vi "Untitled 11.vi"() -> ()   [LabVIEW 2017]
uses:
  <vilib>/Utility/file.llb/Read Delimited Spreadsheet (string).vi
panel:
  out "Array":string[](array[string])
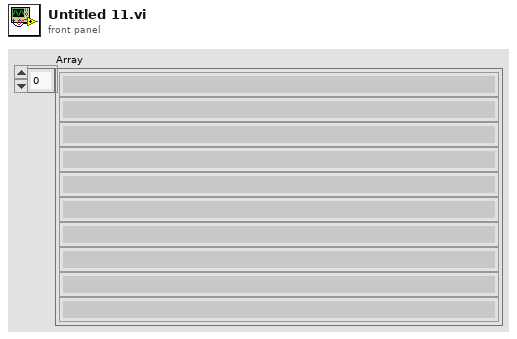
[diagram p1: front panel]
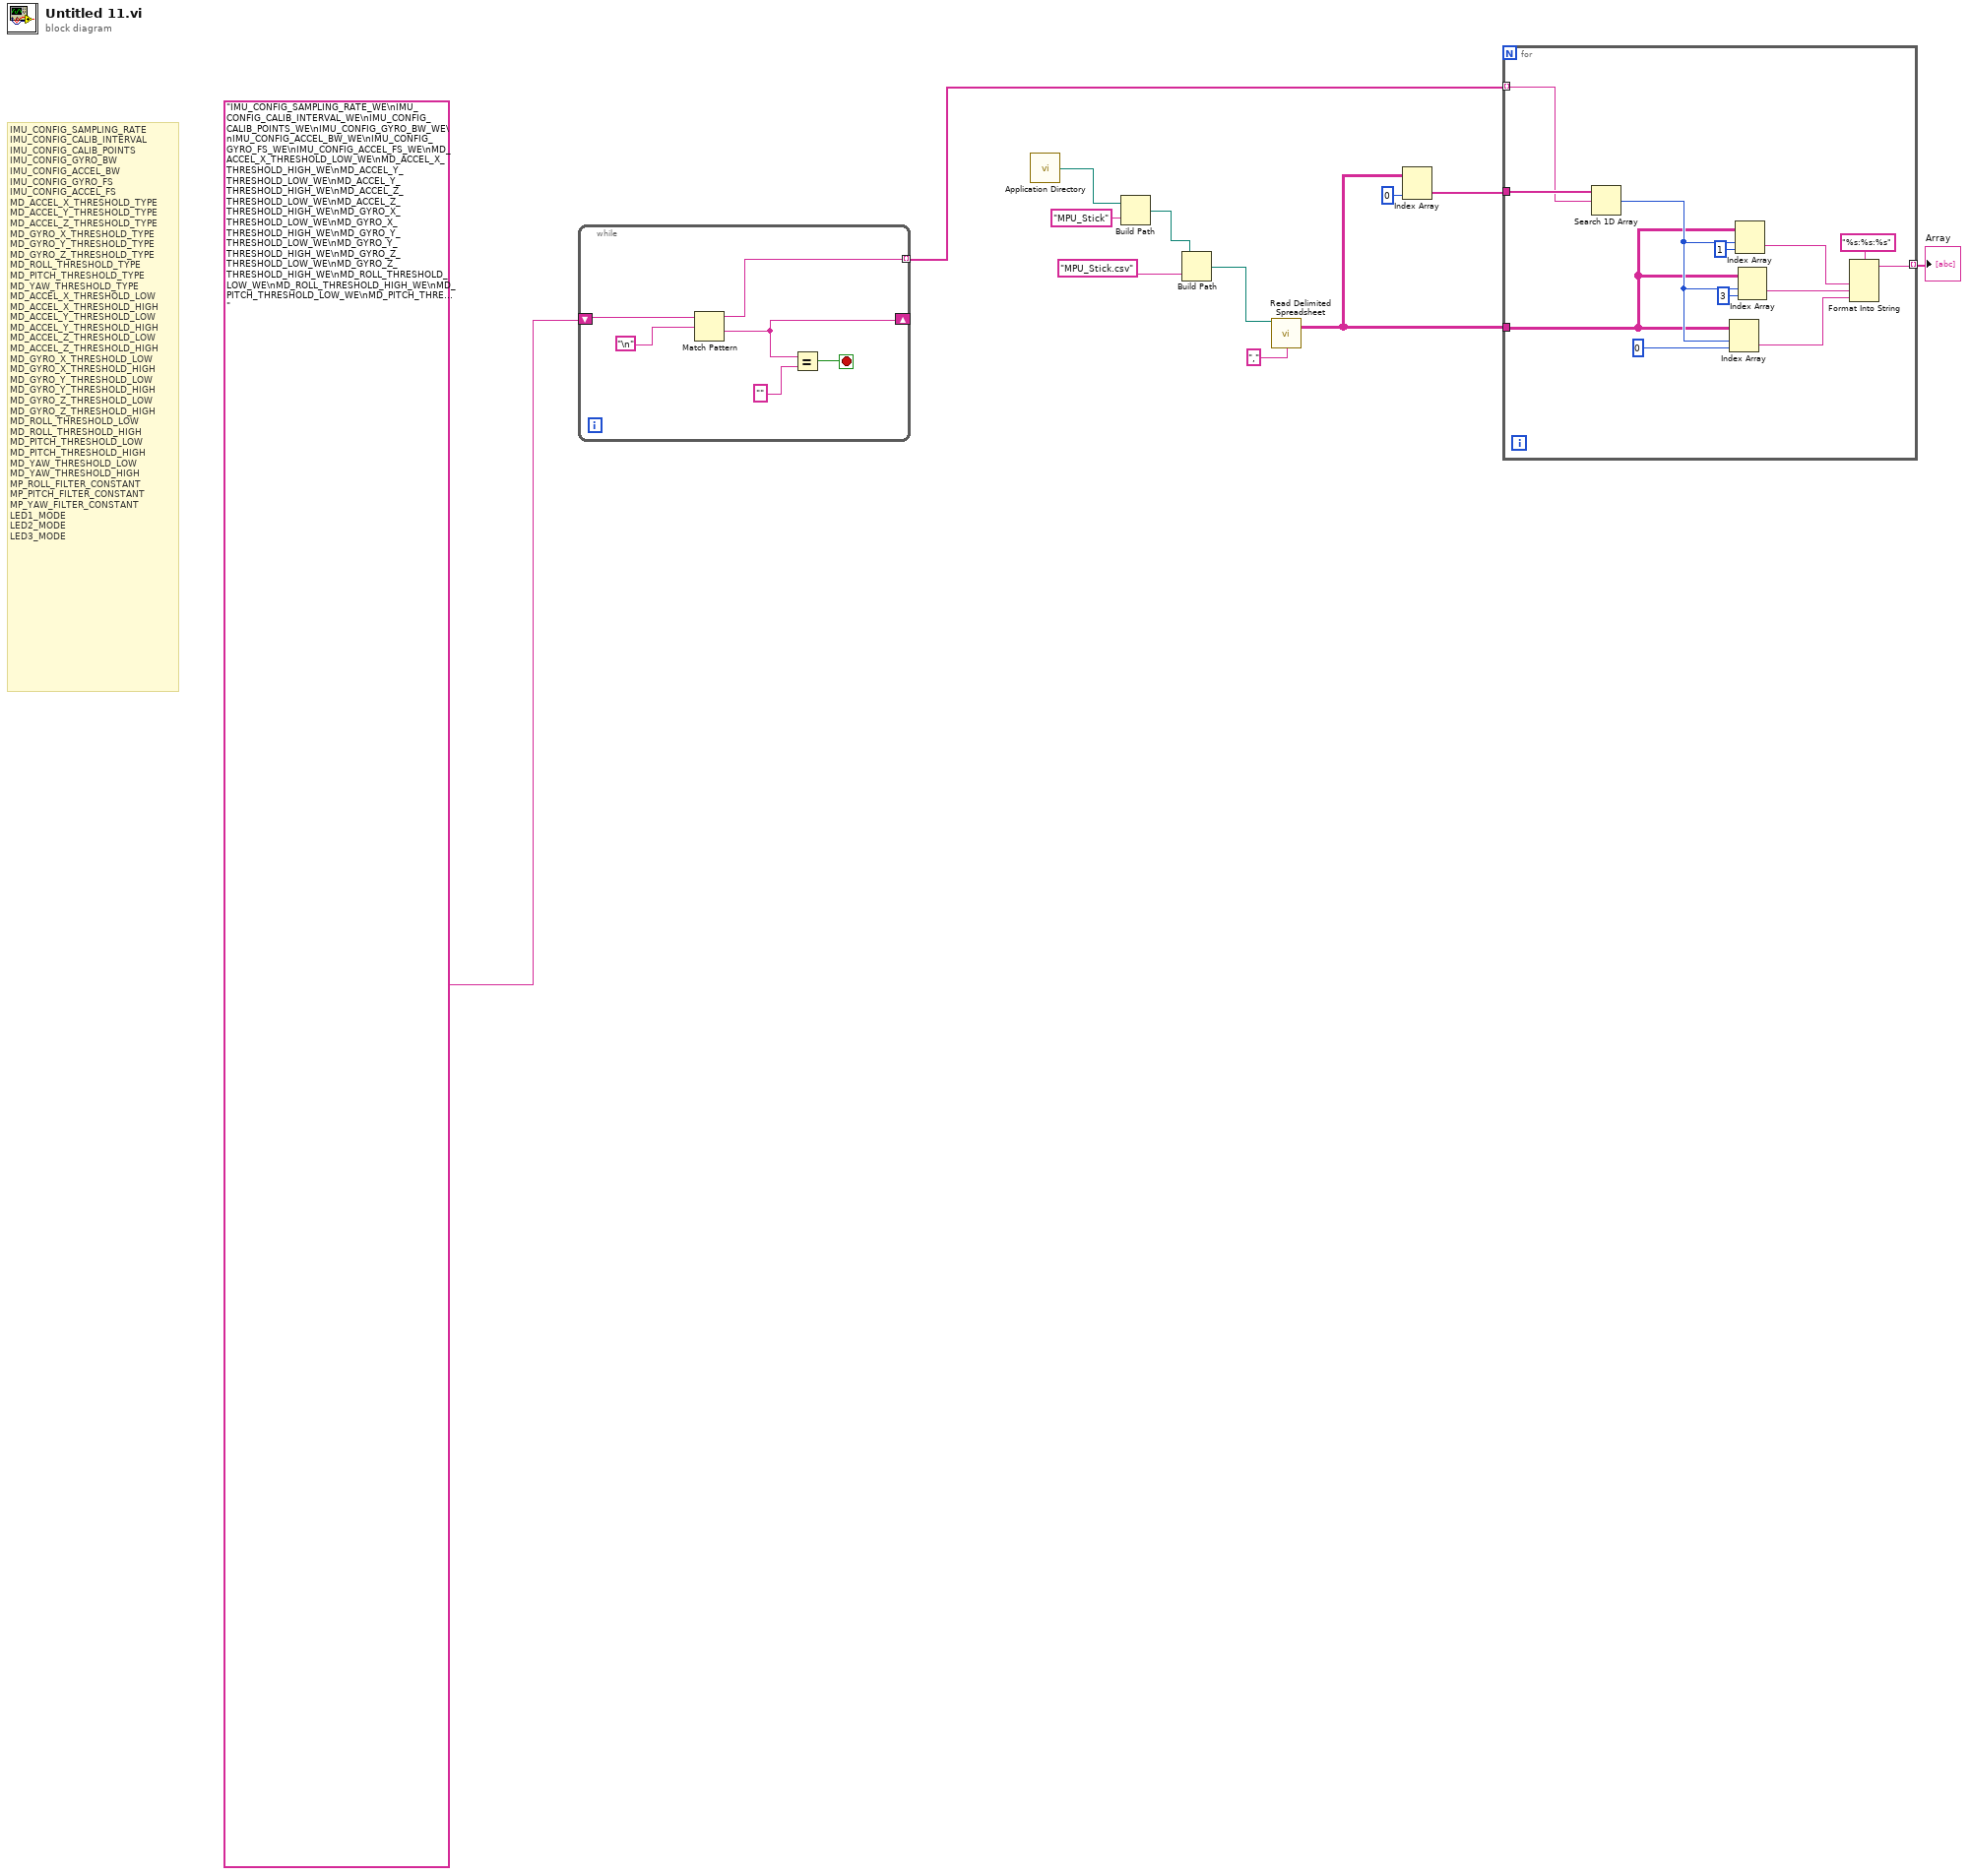
[diagram p0: block diagram]
diagram:
  # "IMU_CONFIG_SAMPLING_RATE\nIMU_CONFIG_CALIB_INTERVAL\nIMU_CONFIG_CALIB_POINTS\nIMU_CONFIG_GYRO_BW\nIMU_CONFIG_ACCEL_BW\nIMU_CONFIG_GYRO_FS\nIMU_CONFIG_ACCEL_FS\nMD_ACCEL_X_THRESHOLD_TYPE\nMD_ACCEL_Y_THRESHOLD_TYPE\nMD_ACCEL_Z_THRESHOLD_TYPE\nMD_GYRO_X_THRESHOLD_TYPE\nMD_GYRO_Y_THRESHOLD_TYPE\nMD_GYRO_Z_THRESHOLD_TYPE\nMD_ROLL_THRESHOLD_TYPE\nMD_PITCH_THRESHOLD_TYPE\nMD_YAW_THRESHOLD_TYPE\nMD_ACCEL_X_THRESHOLD_LOW\nMD_ACCEL_X_THRESHOLD_HIGH\nMD_ACCEL_Y_THRESHOLD_LOW\nMD_ACCEL_Y_THRESHOLD_HIGH\nMD_ACCEL_Z_THRESHOLD_LOW\nMD_ACCEL_Z_THRESHOLD_HIGH\nMD_GYRO_X_THRESHOLD_LOW\nMD_GYRO_X_THRESHOLD_HIGH\nMD_GYRO_Y_THRESHOLD_LOW\nMD_GYRO_Y_THRESHOLD_HIGH\nMD_GYRO_Z_THRESHOLD_LOW\nMD_GYRO_Z_THRESHOLD_HIGH\nMD_ROLL_THRESHOLD_LOW\nMD_ROLL_THRESHOLD_HIGH\nMD_PITCH_THRESHOLD_LOW\nMD_PITCH_THRESHOLD_HIGH\nMD_YAW_THRESHOLD_LOW\nMD_YAW_THRESHOLD_HIGH\nMP_ROLL_FILTER_CONSTANT\nMP_PITCH_FILTER_CONSTANT\nMP_YAW_FILTER_CONSTANT\nLED1_MODE\nLED2_MODE\nLED3_MODE"
  n1 = while {
    shift-right: [w15] -> _
    shift-left: "IMU_CONFIG_SAMPLING_RATE_WE\nIMU_CONFIG_CALIB_INTERVAL_WE\nIMU_CONFIG_CALIB_POINTS_WE\nIMU_CONFIG_GYRO_BW_WE\nIMU_CONFIG_ACCEL_BW_WE\nIMU_CONFIG_GYRO_FS_WE\nIMU_CONFIG_ACCEL_FS_WE\nMD_ACCEL_X_THRESHOLD_LOW_WE\nMD_ACCEL_X_THRESHOLD_HIGH_WE\nMD_ACCEL_Y_THRESHOLD_LOW_WE\nMD_ACCEL_Y_THRESHOLD_HIGH_WE\nMD_ACCEL_Z_THRESHOLD_LOW_WE\nMD_ACCEL_Z_THRESHOLD_HIGH_WE\nMD_GYRO_X_THRESHOLD_LOW_WE\nMD_GYRO_X_THRESHOLD_HIGH_WE\nMD_GYRO_Y_THRESHOLD_LOW_WE\nMD_GYRO_Y_THRESHOLD_HIGH_WE\nMD_GYRO_Z_THRESHOLD_LOW_WE\nMD_GYRO_Z_THRESHOLD_HIGH_WE\nMD_ROLL_THRESHOLD_LOW_WE\nMD_ROLL_THRESHOLD_HIGH_WE\nMD_PITCH_THRESHOLD_LOW_WE\nMD_PITCH_THRESHOLD_HIGH_WE\nMD_YAW_THRESHOLD_LOW_WE\nMD_YAW_THRESHOLD_HIGH_WE\nMP_ROLL_FILTER_CONSTANT_WE\nMP_PITCH_FILTER_CONSTANT_WE\nMP_YAW_FILTER_CONSTANT_WE\nMD_ACCEL_X_THRESHOLD_TYPE_WE\nMD_ACCEL_Y_THRESHOLD_TYPE_WE\nMD_ACCEL_Z_THRESHOLD_TYPE_WE\nMD_GYRO_X_THRESHOLD_TYPE_WE\nMD_GYRO_Y_THRESHOLD_TYPE_WE\nMD_GYRO_Z_THRESHOLD_TYPE_WE\nMD_ROLL_THRESHOLD_TYPE_WE\nMD_PITCH_THRESHOLD_TYPE_WE\nMD_YAW_THRESHOLD_TYPE_WE\nLED1_MODE_WE\nLED2_MODE_WE\nLED3_MODE_WE\nLED_UC_STATE_WE\nLED_UC_DUTY_WE" -> [w18]
    tunnel: [w16] -> w4 mode=indexing
    stop <- w13 stop-if-true
    n2 = Match Pattern(string=w18, regular expression="\n") -> (before substring=w16:string, after substring=w15:string)  [unwired: 1 in, 2 out]
    n3 = Equal?(x=w15, y="") -> (x = y?=w13:bool)
  }
  n4 = call <vilib>:"Application Directory.vi"() -> ("Application Directory"=w11:path)
  n5 = Build Path(base path=w11, name or relative path="MPU_Stick") -> (appended path=w9:path)
  n6 = Build Path(base path=w9, name or relative path="MPU_Stick.csv") -> (appended path=w7:path)
  n7 = call-poly <vilib>:"Read Delimited Spreadsheet.vi"("file path (dialog if empty)"=w7, "delimiter (\\t)"="," ("delimiter (\\t)")) -> ("all rows"=w2:string[][])  [unwired: 8 in, 5 out]
  n8 = Index Array(array=w2, index (col)=0 ("disabled index (col)")) -> (element=w3:string[])  [unwired: 1 in]
  n9 = for {
    tunnel: w4 -> [w29] mode=indexing
    tunnel: w3 -> [w30]
    tunnel: w2 -> [w24]
    tunnel: [w19] -> w1 mode=indexing
    n10 = Search 1D Array(1D array=w30, element=w29) -> (index of element=w25:i32)  [unwired: 1 in]
    n11 = Index Array(array=w24, index (row)=w25, index (col)=0 ("disabled index (col)")) -> (element=w20:string)
    n12 = Index Array(array=w24, index (row)=w25, index (col)=1 ("disabled index (col)")) -> (element=w22:string)
    n13 = Index Array(array=w24, index (row)=w25, index (col)=3 ("disabled index (col)")) -> (element=w21:string)
    n14 = Format Into String(format string="%s:%s:%s", w22, w21, w20) -> (resulting string=w19:string)  [unwired: 2 in, 1 out]
  }
  "Array" <- w1
